vi "寻找满足亮度范围的起始点和终止点.vi"(5 "Color":u32(colorbox)=6618880, 6 "亮度范围":cluster{"下限":dbl, "上限":dbl}={"下限"=0.0, "上限"=100.0}, 7 "亮度均值":dbl[](array[numeric]), 8 "图像矩形框":dbl[](array[numeric]), 9 "引用句柄输入":T1) -> (0 "新的搜索矩形框":dbl[](array[numeric]), 1 "间距1":i32, 2 "亮度均值截取数组":dbl[](array[numeric]), 3 "无异常":bool)   [LabVIEW 2014]
uses:
  <vilib>/vision/Image Controls.llb/IMAQ Image.ctl
panel:
  out "数值":i32
  out "结束行":i32
  out "起始行":i32
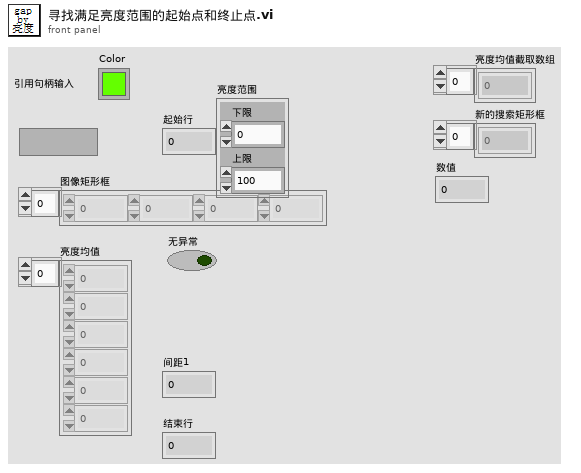
[diagram p1: front panel]
types:
  T1 = typedef "IMAQ Image.ctl" = refnum<image>
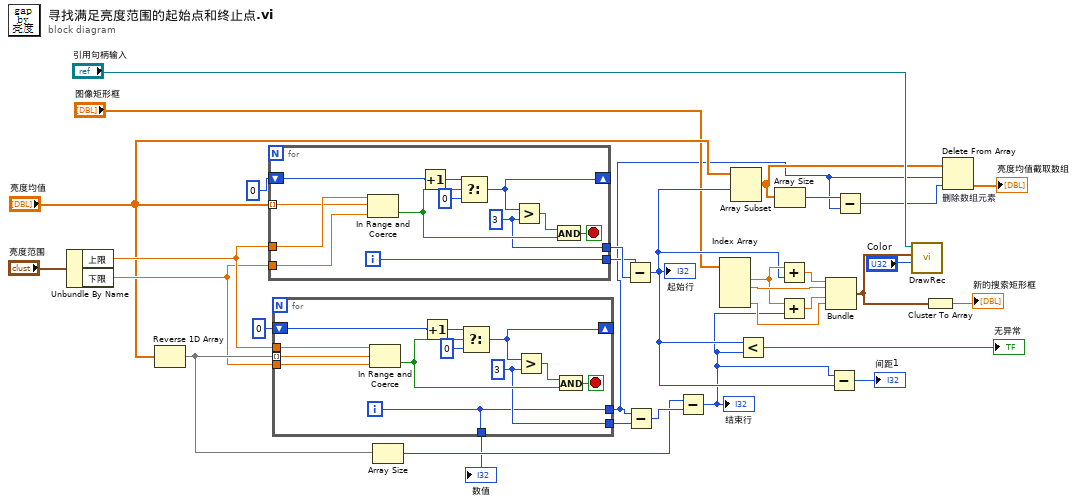
[diagram p0: block diagram]
diagram:
  n1 = Unbundle By Name("亮度范围") -> ("上限"=w16:dbl, "下限"=w15:dbl)
  n2 = Reverse 1D Array(array="亮度均值") -> (reversed array=w20:dbl[])
  n3 = for {
    tunnel: "亮度均值" -> [w33] mode=indexing
    shift-right: [w41] -> _
    shift-left: 0 -> [w43]
    tunnel: [w37] -> w28
    tunnel: [w36] -> w29
    tunnel: w16 -> [w35]
    tunnel: w15 -> [w34]
    i -> [w37]
    stop <- w39 stop-if-true
    w36 = 3 ("y")
    n4 = In Range and Coerce(upper limit=w35, x=w33, lower limit=w34) -> (In Range?=w40:bool)  [unwired: 1 out]
    n5 = Increment(x=w43) -> (x+1=w44:i32)
    n6 = Select(t=w44, s=w40, f=0) -> (s? t:f=w41:i32)
    n7 = Greater?(x=w41, y=w36) -> (0:w42:bool)
    n8 = And(x=w42, y=w40) -> (x .and. y?=w39:bool)
  }
  n9 = for {
    tunnel: w20 -> [w48] mode=indexing
    shift-right: [w53] -> _
    shift-left: 0 ("f") -> [w55]
    tunnel: [w45] -> w2
    tunnel: [w49] -> w30
    tunnel: w16 -> [w47]
    tunnel: w15 -> [w46]
    tunnel: [w45] -> w5
    i -> [w45]
    stop <- w51 stop-if-true
    w49 = 3 ("y")
    n10 = In Range and Coerce(upper limit=w47, x=w48, lower limit=w46) -> (In Range?=w52:bool)  [unwired: 1 out]
    n11 = Increment(x=w55) -> (x+1=w56:i32)
    n12 = Select(t=w56, s=w52, f=0) -> (s? t:f=w53:i32)
    n13 = Greater?(x=w53, y=w49) -> (0:w54:bool)
    n14 = And(x=w54, y=w52) -> (x .and. y?=w51:bool)
  }
  "数值" <- w5
  n15 = Array Size(array=w20) -> (size(s)=w21:i32)
  n16 = Subtract(x=w28, y=w29) -> (x-y=w14:i32)
  "起始行" <- w14
  n17 = Subtract(x=w2, y=w30) -> (x-y=w31:i32)
  n18 = Subtract(x=w21, y=w31) -> (x-y=w12:i32)
  "结束行" <- w12
  n19 = Index Array(array="图像矩形框") -> (element #1=w22:dbl, element #2=w25:dbl, element #4=w26:dbl)  [unwired: 4 in, 1 out]
  n20 = Array Subset(array="亮度均值", index=w14) -> (w4:dbl[])  [unwired: 1 in]
  n21 = Less?(x=w14, y=w12) -> (x < y?=→"无异常":bool)
  n22 = Array Size(array=w4) -> (size(s)=w3:i32)
  n23 = Add(x=w22, y=w14) -> (x+y=w24:dbl)
  n24 = Add(x=w22, y=w12) -> (x+y=w23:dbl)
  n25 = Bundle(w24, w25, w23, w26) -> (w8:cluster{dbl, dbl, dbl, dbl})  [unwired: 1 in]
  n26 = Subtract(x=w12, y=w14) -> (x-y=→"间距1":i32)
  n27 = Subtract(x=w3, y=w2) -> (x-y=w1:i32)
  n28 = call "DrawRec.vi"("Color"="Color", "Rectangle"=w8, "Image"="引用句柄输入") -> ()  [unwired: 8 in, 1 out]
  n29 = Cluster To Array(cluster=w8) -> (array=→"新的搜索矩形框":dbl[])
  n30 = Delete From Array "删除数组元素"(array=w4, length=w2, index=w1) -> (array with subset deleted=→"亮度均值截取数组":dbl[])  [unwired: 1 out]
